vi "BiquadFilter.vi"(0 "x":fxp<+/-,32,14>, 1 "reset":bool=TRUE, 5 "b0":fxp<+/-,32,2>, 7 "b1":fxp<+/-,32,2>, 9 "b2":fxp<+/-,32,2>, 11 "input valid":bool=TRUE, 12 "-a1":fxp<+/-,32,2>, 13 "-a2":fxp<+/-,32,2>) -> (4 "y":fxp<+/-,32,14>, 15 "output valid":bool)   [LabVIEW 2018]
doc: "One second order section, Direct form 1\nRequires 10 cycles per actual sample"
uses:
  <vilib>/rvi/FXPMathLib/FxpMul/XNode/nifxpmath_Multiplier.xnode
  <vilib>/rvi/FXPMathLib/FxpAdd/XNode/nifxpmath_Add.xnode
  <vilib>/rvi/FXPMathLib/sim/FxpSim.dll
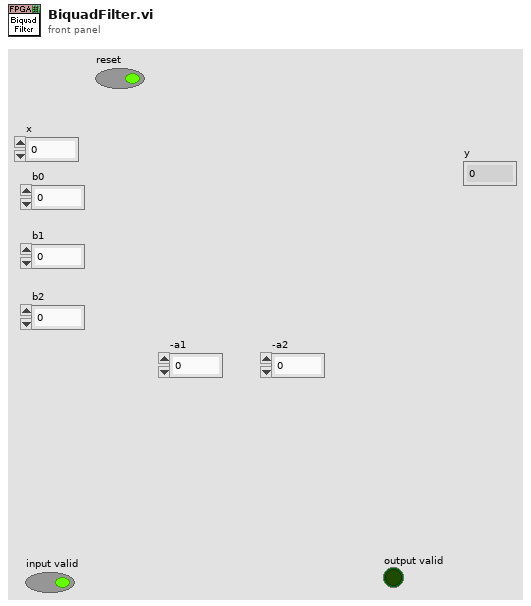
[diagram p1: front panel]
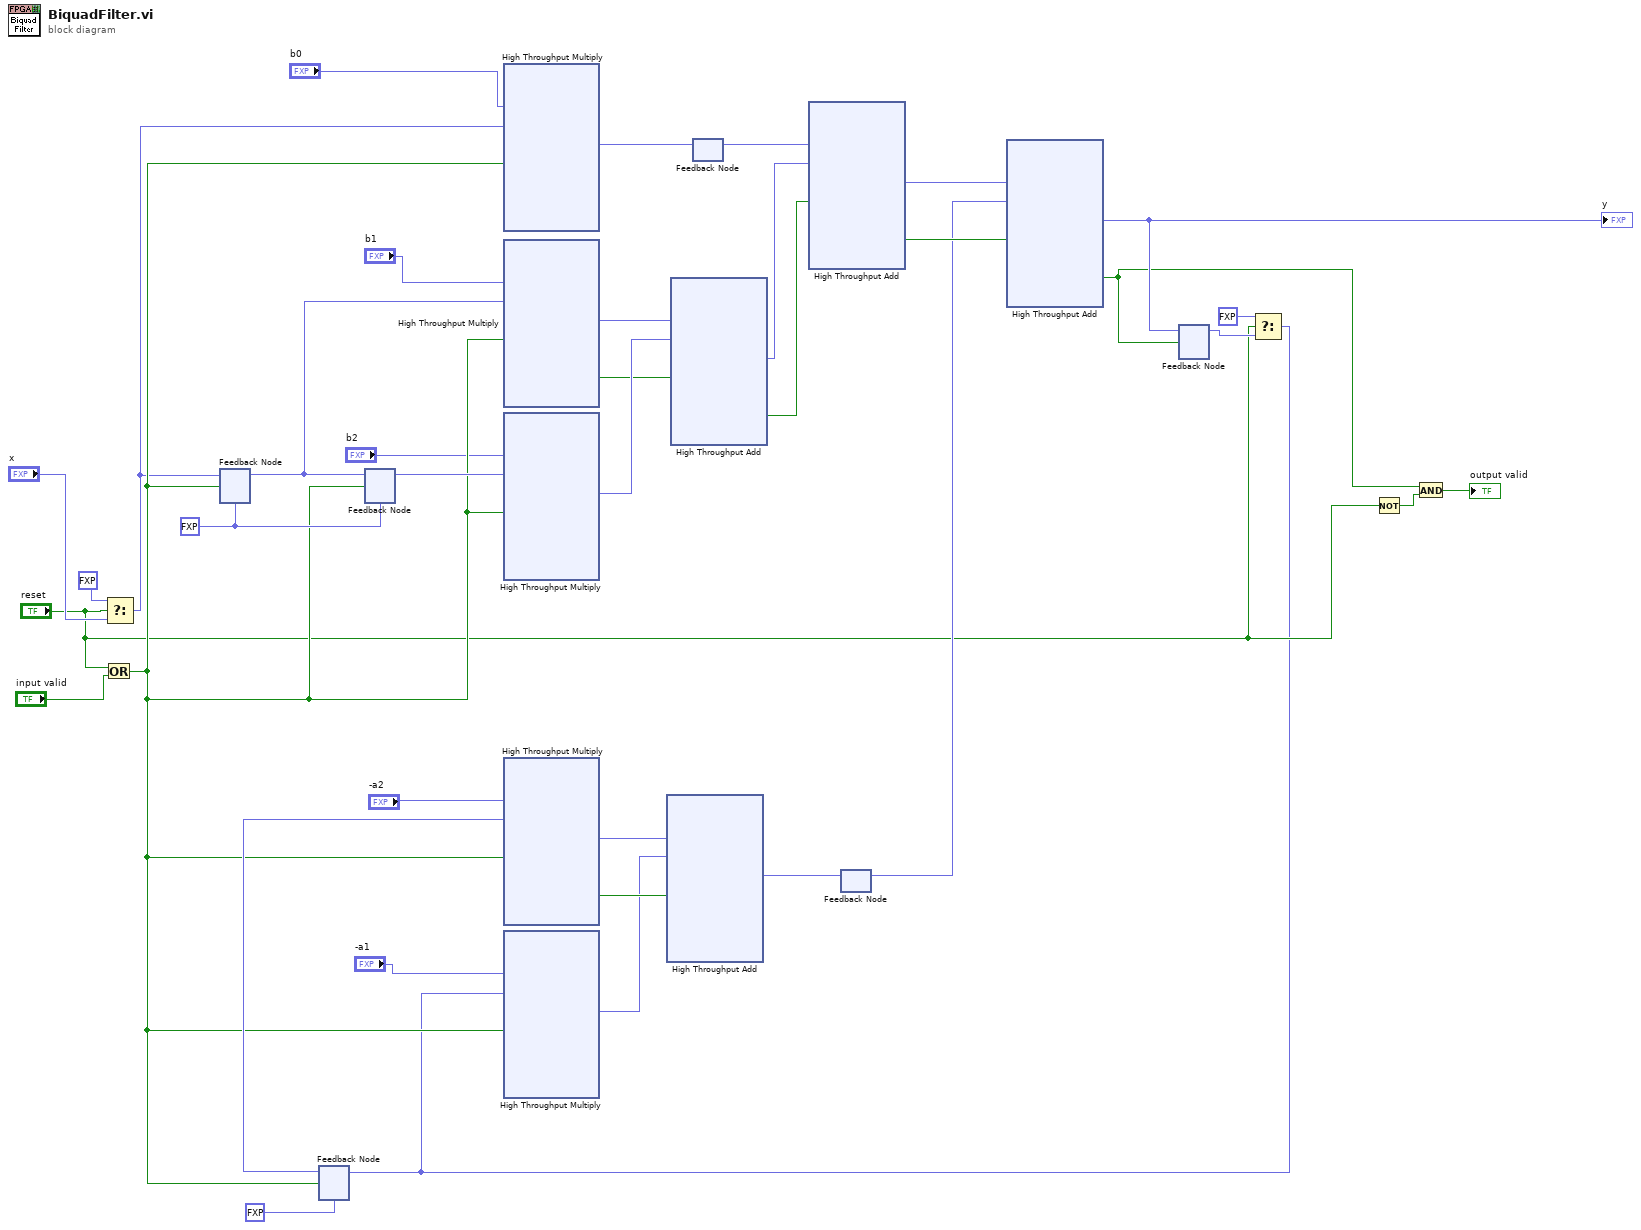
[diagram p0: block diagram]
diagram:
  w21 = fxp<+/-,32,14> 0.0 ("x")
  n1 = Or(x="reset", y="input valid") -> (x .or. y?=w14:bool)
  n2 = Select(t=fxp<+/-,32,14> 0.0 ("x"), s="reset", f="x") -> (s? t:f=w10:fxp<+/-,32,14>)
  n3 = feedback #1(w21) -> (w37:fxp<+/-,32,14>)
  n4 = feedback-in #1(w10, w14) -> ()
  n5 = feedback #2(fxp<+/-,32,14> 0.0 ("x")) -> (w30:fxp<+/-,32,14>)
  n6 = feedback #3(w21) -> (w36:fxp<+/-,32,14>)
  n7 = feedback-in #3(w37, w14) -> ()
  n8 = xnode ("High Throughput Multiply")("x"="b0", "y"=w10, "input valid"=w14) -> ("x*y"=w24:fxp<+/-,32,14>)  [unwired: 1 in, 2 out]
  n9 = xnode ("High Throughput Multiply")("x"="b1", "y"=w37, "input valid"=w14) -> ("x*y"=w35:fxp<+/-,32,14>, "output valid"=w33:bool)  [unwired: 1 in, 1 out]
  n10 = xnode ("High Throughput Multiply")("x"="b2", "y"=w36, "input valid"=w14) -> ("x*y"=w34:fxp<+/-,32,14>)  [unwired: 1 in, 2 out]
  n11 = xnode ("High Throughput Multiply")("x"="-a2", "y"=w30, "input valid"=w14) -> ("x*y"=w29:fxp<+/-,32,14>, "output valid"=w28:bool)  [unwired: 1 in, 1 out]
  n12 = xnode "High Throughput Add"("x"=w35, "y"=w34, "input valid"=w33) -> ("x+y"=w32:fxp<+/-,32,14>, "output valid"=w31:bool)  [unwired: 1 in, 1 out]
  n13 = feedback-in #4(w24) -> ()
  n14 = feedback #4() -> (w23:fxp<+/-,32,14>)  [unwired: 1 in]
  n15 = xnode "High Throughput Add"("x"=w23, "y"=w32, "input valid"=w31) -> ("x+y"=w26:fxp<+/-,32,14>, "output valid"=w25:bool)  [unwired: 1 in, 1 out]
  n16 = feedback #5() -> (w18:fxp<+/-,32,14>)  [unwired: 1 in]
  n17 = xnode "High Throughput Add"("x"=w26, "y"=w18, "input valid"=w25) -> ("x+y"=w19:fxp<+/-,32,14>, "output valid"=w13:bool)  [unwired: 1 in, 1 out]
  "y" <- w19
  n18 = feedback #6() -> (w9:fxp<+/-,32,14>)  [unwired: 1 in]
  n19 = feedback-in #6(w19, w13) -> ()
  n20 = Select(t=fxp<+/-,32,14> 0.0, s="reset", f=w9) -> (s? t:f=w6:fxp<+/-,32,14>)
  n21 = feedback-in #2(w6, w14) -> ()
  n22 = xnode ("High Throughput Multiply")("x"="-a1", "y"=w6, "input valid"=w14) -> ("x*y"=w27:fxp<+/-,32,14>)  [unwired: 1 in, 2 out]
  n23 = xnode "High Throughput Add"("x"=w29, "y"=w27, "input valid"=w28) -> ("x+y"=w22:fxp<+/-,32,14>)  [unwired: 1 in, 2 out]
  n24 = feedback-in #5(w22) -> ()
  n25 = Not(x="reset") -> (.not. x?=w12:bool)
  n26 = And(x=w13, y=w12) -> (x .and. y?=→"output valid":bool)
